vi "Time Until Next Housekeep.vi"(11 "CIFCorePlugin in":refnum<class "CIFCorePlugin.lvclass">) -> (1 "Timeout Valid":bool, 2 "Time Until Next Housekeep (ms)":i32, 3 "Next Housekeep Times":T1, 5 "Housekeep Now":bool)   [LabVIEW 2021, in "CIFCorePlugin.lvclass"]
doc: "This calculates the remaining time before the next scheduled housekeeping (assuming housekeeping is 200ms interval).\nThis is normally used to control the timeout setting for blocking calls such as waiting on new data from a driver. \n\nThe housekeep now indicates the call should be skipped and go directly to housekeeping (will be true when time to next housekeeping is 0).\n\nThe Timeout Valid can be used for tracking statistics on timeouts from blocking calls. It will be valid if the time until next housekeeping is more than 1/2 the housekeeping interval (100ms)."
uses:
  CIFCorePlugin.lvclass
  Typedef/Next Housekeep Times.ctl
  CIFCorePlugin.lvclass/CIFCorePlugin.ctl
  <vilib>/CIF Foundation/CIF Utilities/Time/System Time/LabVIEW Time to TAI Time.vi
  <vilib>/CIF Foundation/CIF Utilities/Time/Time_CIF_U.lvlib
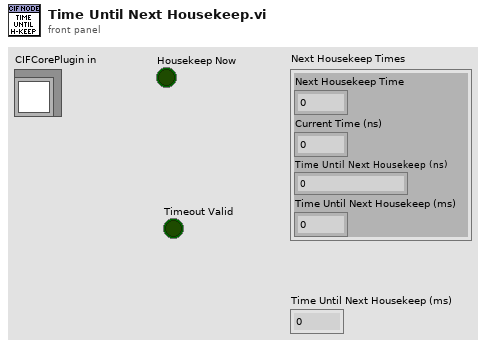
[diagram p1: front panel]
types:
  T1 = typedef "CIFCorePlugin.lvclass/Next Housekeep Times.ctl" = cluster{"Next Housekeep Time":i64, "Current Time (ns)":i64, "Time Until Next Housekeep (ns)":i64, "Time Until Next Housekeep (ms)":i64}
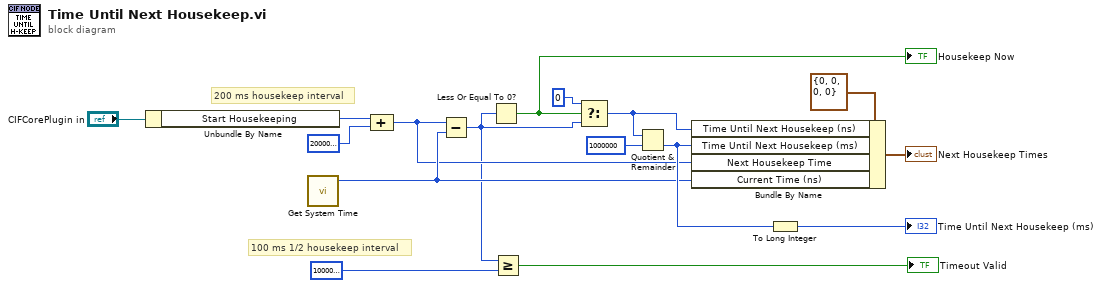
[diagram p0: block diagram]
diagram:
  # "100 ms 1/2 housekeep interval"
  # "200 ms housekeep interval"
  n1 = Unbundle By Name("CIFCorePlugin in") -> ("Start Housekeeping"=w15:i64)
  n2 = call <vilib>:"Get System Time.vi"() -> ("Time (ns)"=w6:i64)  [unwired: 5 in]
  n3 = Compound Arithmetic op=ADD(w15, i64 200000000 ("value")) -> (w5:i64)
  n4 = Subtract(x=w5, y=w6) -> (x-y=w3:i64)
  n5 = Less Or Equal To 0?(x=w3) -> (x <= 0?=w12:bool)
  "Housekeep Now" <- w12
  n6 = Greater Or Equal?(x=w3, y=i64 100000000 ("value")) -> (x >= y?=→"Timeout Valid":bool)
  n7 = Select(t=i64 0, s=w12, f=w3) -> (s? t:f=w9:i64)
  n8 = Quotient & Remainder(x=w9, y=i64 1000000) -> (floor(x/y)=w8:i64)  [unwired: 1 out]
  n9 = Bundle By Name(cluster=T1 {"Next Housekeep Time"=0, "Current Time (ns)"=0, "Time Until Next Housekeep (ns)"=0, "Time Until Next Housekeep (ms)"=0} ("Next Housekeep Times"), "Time Until Next Housekeep (ns)"=w9, "Time Until Next Housekeep (ms)"=w8, "Next Housekeep Time"=w5, "Current Time (ns)"=w6) -> (→"Next Housekeep Times":T1)
  n10 = To Long Integer(number=w8) -> (32bit integer=→"Time Until Next Housekeep (ms)":i32)
